vi "ALTS-2015 Scan Serial Number.vi"(8 "error in":errorcluster, 11 "Serial Number":string) -> (0 "error out":errorcluster, 3 "Valid?":bool)   [LabVIEW 2013]
doc: "Copyright © 2005, Soliton Technologies.\nAll rights reserved."
uses:
  Controls/ALTS-2015 DB Driver Options.ctl
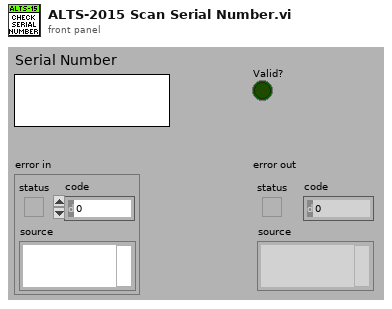
[diagram p1: front panel]
types:
  T1 = typedef "ALTS-2015 DB Driver Options.ctl" = enum16{"Init", "Read DB", "Close"}
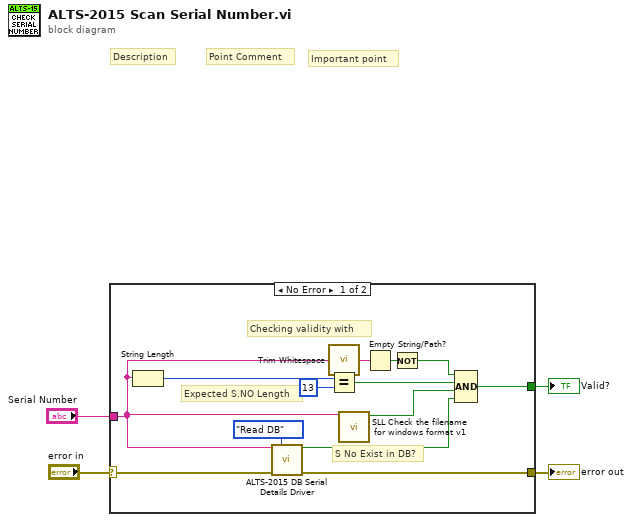
[diagram p0: block diagram]
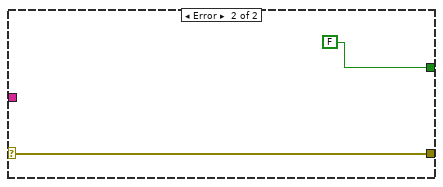
[diagram p2: hidden frame]
diagram:
  # "Important point"
  # "Point Comment"
  # "Description"
  n1 = case shown="No Error" "error in" {
    selector: "error in" -> [w9 w19]
    tunnel: "Serial Number" -> [w7 _]
    tunnel: [w8 w19] -> w3
    tunnel: [w12 FALSE] -> w1
    frame No Error {
      # "S No Exist in DB?"
      # "Checking validity with"
      # "Expected S.NO Length"
      n2 = String Length(string=w7) -> (length=w15:i32)
      n3 = call "ALTS-2015 DB Serial Details Driver.vi"("Serial Number"=w7, "Operation"=ALTS-2015_DB_Driver_Options."Read DB", "error in (no error)"=w9) -> ("S No Valid?"=w5:bool, "error out"=w8:errorcluster)  [unwired: 10 in, 1 out]
      n4 = call <vilib>:"Trim Whitespace.vi"("string"=w7) -> ("trimmed string"=w17:string)  [unwired: 1 in]
      n5 = Equal?(x=w15, y=13) -> (x = y?=w13:bool)
      n6 = call "SLL Check the filename for windows format v1.vi"("File Name"=w7) -> ("File Name OK?"=w11:bool)  [unwired: 10 in]
      n7 = Empty String/Path?(string/path=w17) -> (empty?=w16:bool)
      n8 = Not(x=w16) -> (.not. x?=w10:bool)
      n9 = Compound Arithmetic op=AND(w10, w13, w11, w5) -> (w12:bool)
    }
    frame Error {
    }
  }
  "error out" <- w3
  "Valid?" <- w1
